vi "ConvertStrToByteArr.vi"(11 "data in":string) -> (3 "arrByte":u8[](array[numeric]))   [LabVIEW 2018, in "Library-DataConvert.lvlib"]
uses:
  Library-DataConvert.lvlib
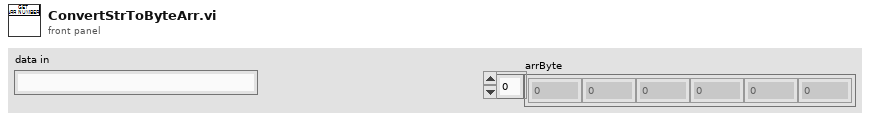
[diagram p1: front panel]
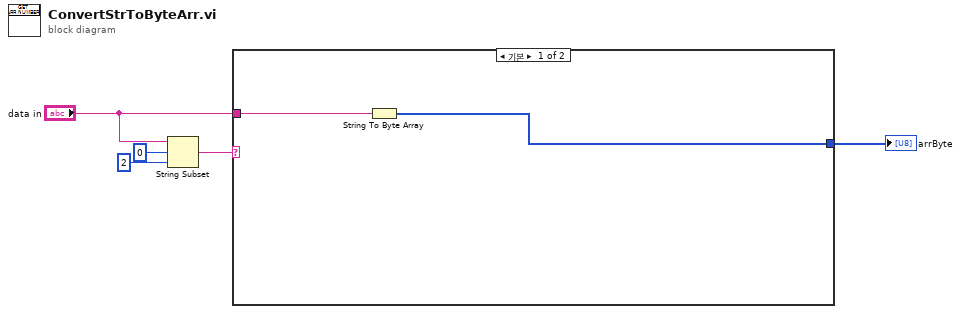
[diagram p0: block diagram]
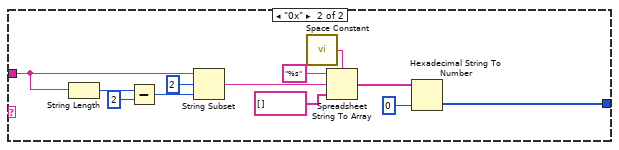
[diagram p2: hidden frame]
diagram:
  n1 = String Subset(string="data in", offset (0)=0 ("오프셋(0)"), length (rest)=2 ("길이(나머지)")) -> (substring=w3:string)
  n2 = case shown="기본" w3 {
    tunnel: "data in" -> [w7 w19]
    tunnel: [w6 w8] -> w1
    frame Default {
      n3 = String To Byte Array(string=w7) -> (unsigned byte array=w6:u8[])
    }
    frame "0x" {
      n4 = String Length(string=w19) -> (length=w17:i32)
      n5 = Subtract(x=w17, y=2) -> (x-y=w15:i32)
      n6 = String Subset(string=w19, offset (0)=2 ("오프셋(0)"), length (rest)=w15) -> (substring=w9:string)
      n7 = call <vilib>:"Space Constant.vi"() -> ("String"=w14:string)
      n8 = Spreadsheet String To Array(delimiter (Tab)=w14, format string="%s" ("포맷 문자열"), spreadsheet string=w9, array type (2D Dbl)=string[] []) -> (array=w12:string[])
      n9 = Hexadecimal String To Number(string=w12, default (0uL)=u8 0) -> (number=w8:u8[])  [unwired: 1 in, 1 out]
    }
  }
  "arrByte" <- w1
